vi "ROI entry-Fire user event-Experiment load.vi"(11 "User Events Cluster":T1) -> (0 "error out":errorcluster)   [LabVIEW 2013]
uses:
  Typedefs/Offsets cluster.ctl
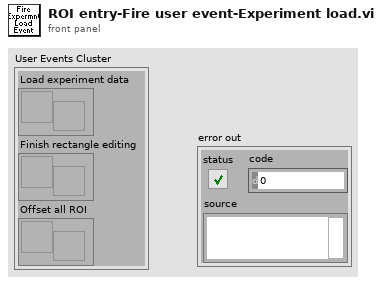
[diagram p1: front panel]
types:
  T1 = cluster{"Load experiment data":refnum<user-event>, "Finish rectangle editing":refnum<user-event>, "Offset all ROI":refnum<user-event>}
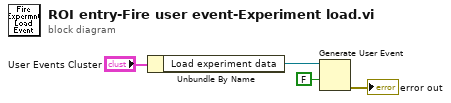
[diagram p0: block diagram]
diagram:
  n1 = Unbundle By Name("User Events Cluster") -> ("Load experiment data"=w4:refnum<user-event>)
  n2 = Generate User Event(user event=w4, event data cluster=FALSE ("event data")) -> (error out=→"error out":errorcluster)  [unwired: 2 in, 1 out]
